vi "IMAQdxGrab.vi"() -> ()   [LabVIEW 2015]
doc: "The Grab VI acquires images continuously and displays the images in an image control using high-level acquisition VIs. A grab is appropriate for high-speed applications in which you need to process only one image at a time."
uses:
  <vilib>/vision/driver/IMAQdx.llb/IMAQdx Attribute Type.ctl
  <vilib>/vision/driver/IMAQdx.llb/IMAQdx Attribute Visibility.ctl
  <vilib>/vision/driver/NI_Vision_Acquisition_Software.lvlib
  <resource>/objmgr/imaqdx.rc
panel:
  out "Array":T1[](array[typedef])
  in  "Stop 2":bool
  out "Frame Rate":dbl(knob) scale=0.0..100.0
  out "Image":T2(plugin-control)
  out "Buffer Number":u32
  in  "Set Attribute":bool
  in  "Attribute Value":string
  in  "Attribute Name":u32(ring) items=["CameraAttributes::Exposure::Mode", "CameraAttributes::Exposure::Value", "CameraAttributes::Gain::Mode", "CameraAttributes::Gain::Value"]
  in  "Camera Name":refnum<k21> caption="IMAQdx Session"
  in  "Stop":bool
  # "Overview: Demonstrates how to acquire images continuously using a Grab acquisition.\nRequirements: Vision Acquisition Software\nInstructions: \n1. Select the Camera Name.\n2. Run the VI"
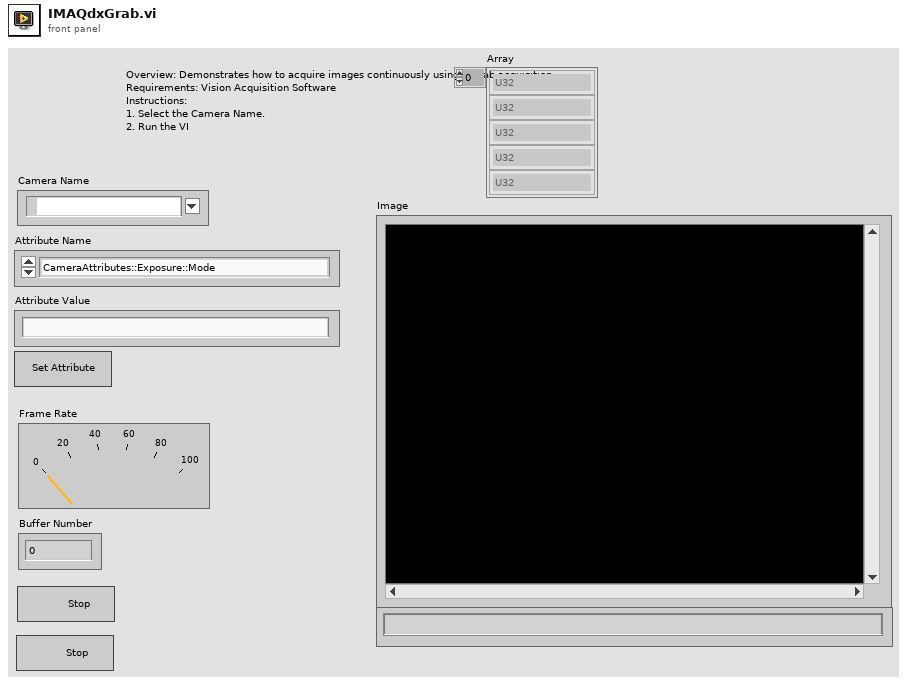
[diagram p1: front panel]
types:
  T1 = typedef "NI_Vision_Acquisition_Software.lvlib/IMAQdx Attribute Type.ctl" = enum32{"U32", "I64", "DBL", "String", "Enum", "Bool", "Command"}
  T2 = typedef "IMAQ Image.ctl" = refnum<image>
  T3 = typedef "NI_Vision_Acquisition_Software.lvlib/IMAQdx Attribute Visibility.ctl" = enum32{"Simple", "Intermediate", "Advanced"}
  T4 = typedef "IMAQdx.ctl" = refnum<k21>
  T5 = cluster{"Attribute Type":T1, "Readable":bool, "Writable":bool, "Attribute Name":string}[]
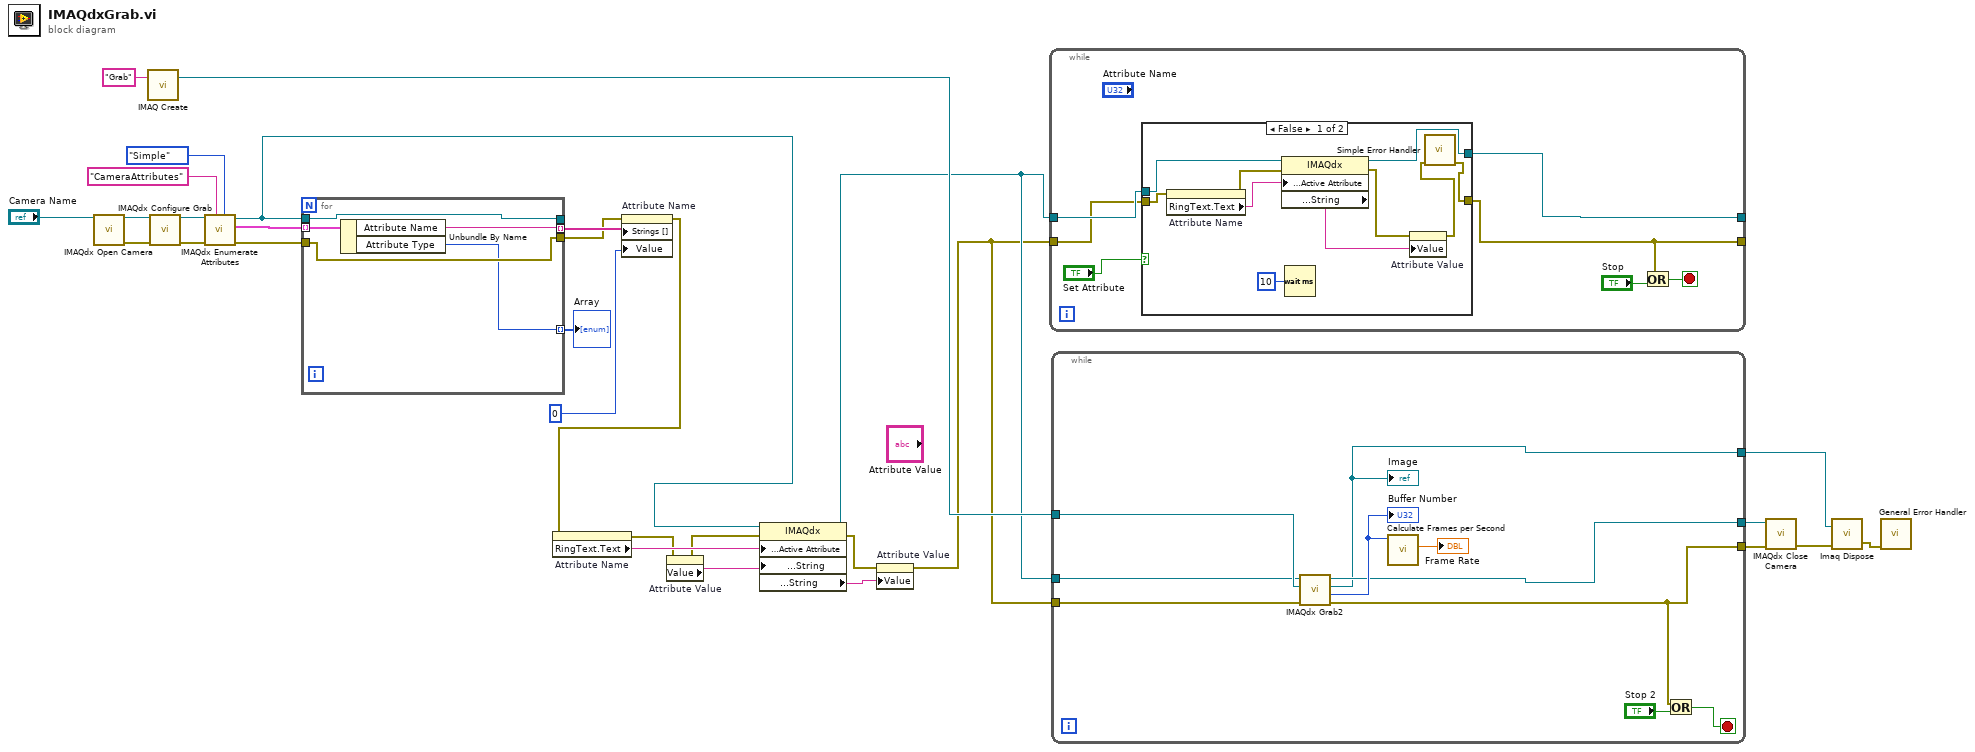
[diagram p0: block diagram]
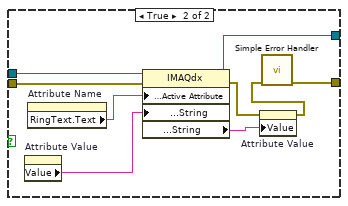
[diagram p2: hidden frame]
diagram:
  n1 = call <vilib>:"IMAQdx Open Camera.vi"("Session In"="Camera Name") -> ("error out"=w30:errorcluster, "Session Out"=w29:T4)  [unwired: 2 in, 7 out]
  n2 = call "IMAQ Create"("Image Name"="Grab") -> ("New Image"=w13:T2)  [unwired: 3 in, 2 out]
  n3 = call <vilib>:"IMAQdx Configure Grab.vi"("error in"=w30, "Session In"=w29) -> ("error out"=w21:errorcluster, "Session Out"=w22:T4)  [unwired: 8 out]
  n4 = call <vilib>:"IMAQdx Enumerate Attributes.vi"("Visibility"=IMAQdx_Attribute_Visibility."Simple", "Root"="CameraAttributes", "error in"=w21, "Session In"=w22) -> ("error out"=w17:errorcluster, "Attribute Information Array"=w20:T5, "Session Out"=w9:T4)  [unwired: 5 out]
  n5 = for {
    tunnel: w20 -> [w35] mode=indexing
    tunnel: [w32] -> w19 mode=indexing
    tunnel: w9 -> [w34]
    tunnel: [w34] -> _
    tunnel: w17 -> [w33]
    tunnel: [w33] -> w2
    tunnel: [w31] -> w1 mode=indexing
    n6 = Unbundle By Name(w35) -> ("Attribute Name"=w32:string, "Attribute Type"=w31:T1)
  }
  "Array" <- w1
  n7 = property on="Attribute Name" class="Ring (strict)"(error in=w2, "Strings []"=w19, "Value"=u32 0 ("BufferInterval")) -> (error out=w5:errorcluster)  [unwired: 1 in, 1 out]
  n8 = property on="Attribute Name" class="Ring (strict)"(error in=w5) -> (error out=w4:errorcluster, "RingText.Text"=w12:string)  [unwired: 1 in, 1 out]
  n9 = property on="Attribute Value" class="Str"(error in=w4) -> (error out=w3:errorcluster, "Value"=w11:string)  [unwired: 1 in, 1 out]
  n10 = property class="IMAQdx"(reference=w9, error in=w3, "Camera Attributes:Active Attribute"=w12, "Camera Attributes:Value:String"=w11) -> (reference out=w8:T4, error out=w7:errorcluster, "Camera Attributes:Value:String"=w10:string)
  n11 = property on="Attribute Value" class="Str"(error in=w7, "Value"=w10) -> (error out=w6:errorcluster)  [unwired: 1 in, 1 out]
  n12 = while {
    tunnel: [w36] -> _
    tunnel: w6 -> [w39]
    tunnel: w8 -> [w40]
    tunnel: [w37] -> _
    stop <- w42 stop-if-true
    n13 = case shown="False" "Set Attribute" {
      tunnel: w40 -> [w49 w61]
      tunnel: [w43 w60] -> w36
      tunnel: [w44 w59] -> w37
      tunnel: w39 -> [w50 w58]
      frame False {
        n14 = property on="Attribute Name" class="Ring (strict)"(error in=w50) -> (error out=w48:errorcluster, "RingText.Text"=w51:string)  [unwired: 1 in, 1 out]
        n15 = property class="IMAQdx"(reference=w49, error in=w48, "Camera Attributes:Active Attribute"=w51) -> (reference out=w43:T4, error out=w47:errorcluster, "Camera Attributes:Value:String"=w46:string)
        n16 = Wait (ms)(milliseconds to wait=u32 10) -> ()  [unwired: 1 out]
        n17 = property on="Attribute Value" class="Str"(error in=w47, "Value"=w46) -> (error out=w45:errorcluster)  [unwired: 1 in, 1 out]
        n18 = call <vilib>:"Simple Error Handler.vi"("error in (no error)"=w45) -> ("error out"=w44:errorcluster)  [unwired: 1 in, 7 out]
      }
      frame True {
        n19 = property on="Attribute Value" class="Str"() -> ("Value"=w56:string)  [unwired: 2 in, 2 out]
        n20 = property on="Attribute Name" class="Ring (strict)"() -> ("RingText.Text"=w55:string)  [unwired: 2 in, 2 out]
        n21 = property class="IMAQdx"(reference=w61, error in=w58, "Camera Attributes:Active Attribute"=w55, "Camera Attributes:Value:String"=w56) -> (reference out=w60:T4, error out=w54:errorcluster, "Camera Attributes:Value:String"=w57:string)
        n22 = property on="Attribute Value" class="Str"(error in=w54, "Value"=w57) -> (error out=w53:errorcluster)  [unwired: 1 in, 1 out]
        n23 = call <vilib>:"Simple Error Handler.vi"("error in (no error)"=w53) -> ("error out"=w59:errorcluster)  [unwired: 1 in, 7 out]
      }
    }
    n24 = Or(x=w37, y="Stop") -> (x .or. y?=w42:bool)
  }
  n25 = while {
    tunnel: [w62] -> w16
    tunnel: [w69] -> w15
    tunnel: [w68] -> w14
    tunnel: w6 -> [w67]
    tunnel: w13 -> [w66]
    tunnel: w8 -> [w65]
    stop <- w63 stop-if-true
    n26 = call <vilib>:"IMAQdx Grab2.vi"("error in"=w67, "Image In"=w66, "Session In"=w65) -> ("error out"=w62:errorcluster, "Buffer Number Out"=w71:u32, "Image Out"=w68:T2, "Session Out"=w69:T4)  [unwired: 5 in]
    "Image" <- w68
    "Buffer Number" <- w71
    n27 = call <vilib>:"Calculate Frames per Second.vi"("Buffer Number"=w71) -> ("Processed Frames/s"=→"Frame Rate":dbl)  [unwired: 8 in, 2 out]
    n28 = Or(x=w62, y="Stop 2") -> (x .or. y?=w63:bool)
  }
  n29 = call <vilib>:"IMAQdx Close Camera.vi"("error in"=w16, "Session In"=w15) -> ("error out"=w27:errorcluster)  [unwired: 9 out]
  n30 = call "Imaq Dispose"("Image"=w14, "error in (no error)"=w27) -> ("error out"=w26:errorcluster)  [unwired: 4 in]
  n31 = call <vilib>:"General Error Handler.vi"("error in (no error)"=w26) -> ()  [unwired: 2 in, 13 out]
